vi "Get Send Method Path.vi"(11 "Message Scripter":refnum<class "Message Scripter.lvclass">) -> (2 "Send Method Path":path)   [LabVIEW 2020, in "Message Maker.lvlib" / "Message Scripter.lvclass"]
uses:
  Message Scripter.lvclass
  Message Maker.lvlib
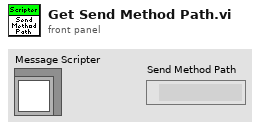
[diagram p1: front panel]
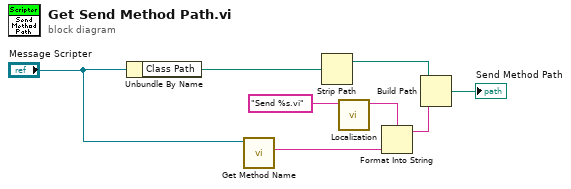
[diagram p0: block diagram]
diagram:
  n1 = Unbundle By Name("Message Scripter") -> ("Class Path"=w5:path)
  n2 = call-dynamic "Get Method Name.vi"("Message Maker in"="Message Scripter") -> ("Method Name"=w2:string)  [unwired: 10 in]
  n3 = Strip Path(path=w5) -> (stripped path=w3:path)  [unwired: 1 out]
  n4 = call "Localization.vi"("Unlocalized"="Send %s.vi") -> ("Localized"=w7:string)  [unwired: 10 in]
  n5 = Format Into String(format string=w7, w2) -> (resulting string=w6:string)  [unwired: 2 in, 1 out]
  n6 = Build Path(base path=w3, name or relative path=w6) -> (appended path=→"Send Method Path":path)
